vi "Ophir_Measure.vi"(0 "INSTR_PARAM 2":refnum<vi>, 1 "error in (no error)":errorcluster) -> (2 "Overrange":bool, 3 "Power,uW":dbl, 4 "error out":errorcluster)   [LabVIEW 2012]
uses:
  Controls/Instr_Param.ctl
  Controls/USB4000_Data.ctl
  <vilib>/Analysis/NI_AALBase.lvlib
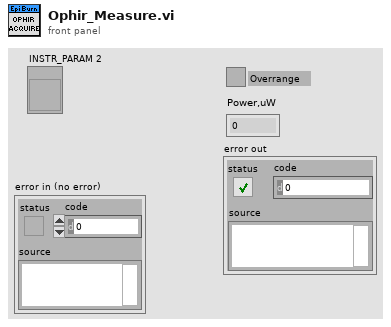
[diagram p1: front panel]
types:
  T1 = typedef "Instr_Param.ctl" = cluster{"Keithley_Param":cluster{"Start Current,mA":dbl, "Stop Current,mA":dbl, "Voltage Compliance,V":dbl, "GPIB":string}, "USB4000_Param":cluster{"Integration Time":i32, "Wl min,nm":dbl, "Wl max,nm":dbl, "USB4000":T2}, "Ophir_Param":cluster{"VISA resource name":refnum<visa-resource-name>, "Calibration Wl":dbl}}
  T2 = typedef "USB4000_Data.ctl" = cluster{"Wrapper Out":u32, "Number of Spectrometers":i32, "Wavelength":dbl[], "EL Spectrum":dbl[], "Int Time (usec)":i32, bool, "Background":dbl[]}
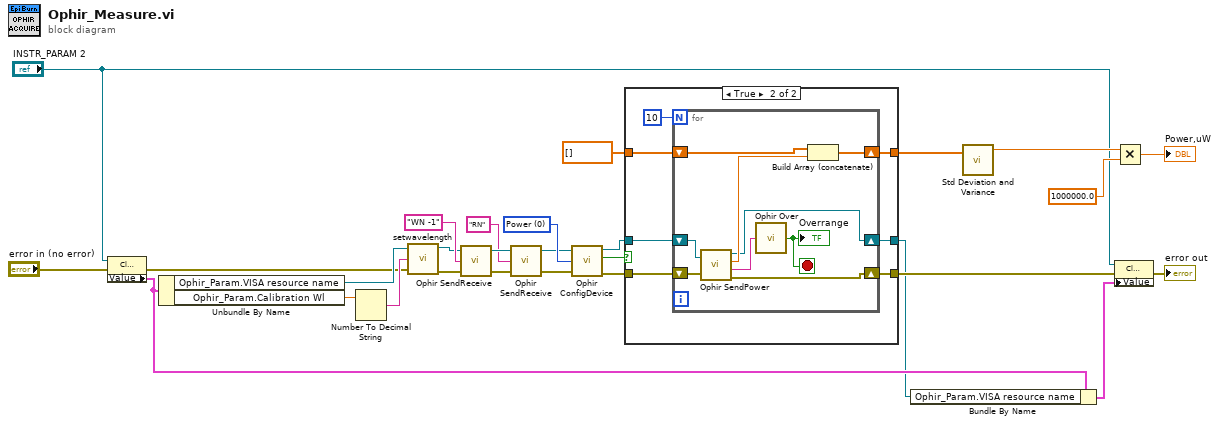
[diagram p0: block diagram]
diagram:
  w22 = u16 0 items=["Power", "Energy", "Frequency"] ("Measure Choice (0:Power)")
  n1 = property class="Clust (strict)"(reference="INSTR_PARAM 2", error in="error in (no error)") -> (error out=w8:errorcluster, "Value"=w3:T1)  [unwired: 1 out]
  n2 = Unbundle By Name(w3) -> ("Ophir_Param.VISA resource name"=w9:refnum<visa-resource-name>, "Ophir_Param.Calibration Wl"=w10:dbl)
  n3 = Number To Decimal String(number=w10) -> (decimal integer string=w11:string)  [unwired: 1 in]
  n4 = call "setwavelength.vi"("Dup Visa Session"=w9, "Set Wavelength"=w11, "error in (no error)"=w8) -> ("dup Visa Session"=w27:refnum<visa-resource-name>, "error out"=w26:errorcluster)  [unwired: 3 in]
  n5 = call "Ophir SendReceive.vi"("error in (no error)"=w26, "Command"="WN -1", "Visa Session"=w27) -> ("error out"=w23:errorcluster, "dup Visa Session"=w25:refnum<visa-resource-name>)  [unwired: 1 out]
  n6 = call "Ophir SendReceive.vi"("error in (no error)"=w23, "Command"="RN", "Visa Session"=w25) -> ("error out"=w20:errorcluster, "dup Visa Session"=w21:refnum<visa-resource-name>)  [unwired: 1 out]
  n7 = call "Ophir ConfigDevice.vi"("Visa Session"=w21, "Measure Choice (0:Power)"=w22, "error in (no error)"=w20) -> ("dup Visa Session"=w17:refnum<visa-resource-name>, "OK ?"=w19:bool, "error out"=w18:errorcluster)  [unwired: 1 out]
  n8 = case shown="True" w19 {
    tunnel: w18 -> [w30 w36]
    tunnel: w17 -> [w31 w37]
    tunnel: dbl[] [] -> [w29 w38]
    tunnel: [w31 w35] -> w2
    tunnel: [w30 w34] -> w4
    tunnel: [w29 w33] -> w15
    frame False {
    }
    frame True {
      n9 = for {
        N: 10 -> [_]
        shift-right: [w41] -> w33
        shift-left: w38 -> [w47]
        shift-right: [w42] -> w35
        shift-left: w37 -> [w45]
        shift-right: [w43] -> w34
        shift-left: w36 -> [w44]
        stop <- w39 stop-if-true
        n10 = call "Ophir SendPower.vi"("Visa Session"=w45, "error in (no error)"=w44) -> ("dup Visa Session"=w42:refnum<visa-resource-name>, "Value Number"=w46:dbl, "Value String"=w40:string, "error out"=w43:errorcluster)
        n11 = call "Ophir Over.vi"("Value String"=w40) -> ("Overrange"=w39:bool)
        "Overrange" <- w39
        n12 = Build Array (concatenate)(w47, w46) -> (w41:dbl[])
      }
    }
  }
  n13 = Bundle By Name(cluster=w3, "Ophir_Param.VISA resource name"=w2) -> (w1:T1)
  n14 = call <vilib>:"Std Deviation and Variance.vi"("X"=w15) -> ("mean"=w13:dbl)  [unwired: 1 in, 2 out]
  n15 = Multiply(x=w13, y=1000000.0) -> (x*y=→"Power,uW":dbl)
  n16 = property class="Clust (strict)"(reference="INSTR_PARAM 2", error in=w4, "Value"=w1) -> (error out=→"error out":errorcluster)  [unwired: 1 out]
